vi "getNe.vi"(6 "plasma,a.m.u.":dbl, 9 "Sprobe, cm^2":dbl, 10 "Te,eV":dbl, 11 "Is(mA)":dbl) -> (3 "Ne,cm^-3":dbl)   [LabVIEW 2014]
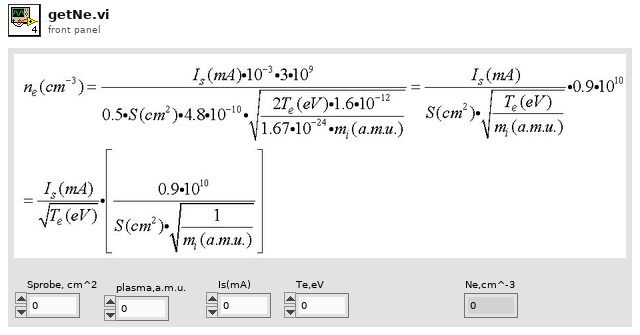
[diagram p1: front panel]
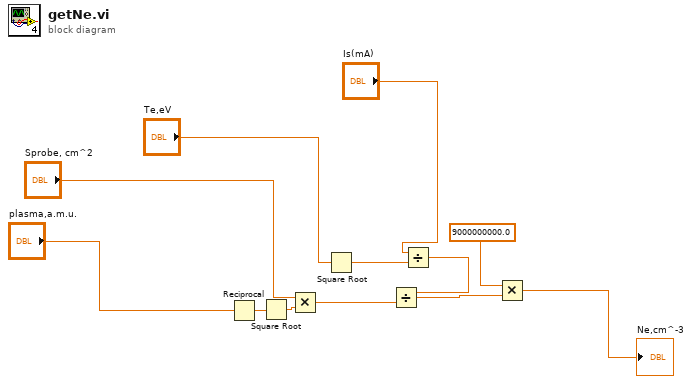
[diagram p0: block diagram]
diagram:
  n1 = Reciprocal(x="plasma,a.m.u.") -> (1/x=w11:dbl)
  n2 = Square Root(x=w11) -> (sqrt(x)=w10:dbl)
  n3 = Multiply(x="Sprobe, cm^2", y=w10) -> (x*y=w8:dbl)
  n4 = Square Root(x="Te,eV") -> (sqrt(x)=w9:dbl)
  n5 = Divide(x="Is(mA)", y=w9) -> (x/y=w7:dbl)
  n6 = Divide(x=w7, y=w8) -> (x/y=w6:dbl)
  n7 = Multiply(x=9000000000.0, y=w6) -> (x*y=→"Ne,cm^-3":dbl)
